vi "MH_GetAllCountRates.vi"(8 "error in (no error)":errorcluster, 10 "cntrates_buf":i32[](array[numeric]), 11 "devidx":i32) -> (0 "error out":errorcluster, 1 "cntrates":i32[](array[numeric]), 2 "syncrate":i32, 3 "return type":i32)   [LabVIEW 2019]
uses:
  <userlib>/MultiHarp150/MH_DllPath_global.vi
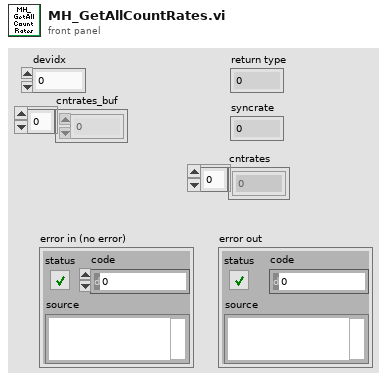
[diagram p1: front panel]
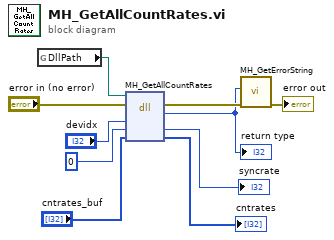
[diagram p0: block diagram]
diagram:
  n1 = global read "MH_DllPath_global.vi" "DllPath"() -> (w9:path)
  n2 = dll-call lib="MHLib64.dll" fn="MH_GetAllCountRates"(path in=w9, error in="error in (no error)", "devidx"="devidx", "syncrate"=0 ("rate"), "cntrates"="cntrates_buf") -> (error out=w7:errorcluster, "return type"=w6:i32, "syncrate"=→"syncrate":i32, "cntrates"=→"cntrates":i32[])  [unwired: 2 in, 1 out]
  "return type" <- w6
  n3 = call <userlib>:"MH_GetErrorString.vi"("error in (no error)"=w7, "code"=w6) -> ("error out"=→"error out":errorcluster)  [unwired: 7 in, 2 out]
